vi "WildBugChilGru_V2.0.0.vi"() -> ()   [LabVIEW 2014]
uses:
  <vilib>/Utility/miscctls.llb/LVPointTypeDef.ctl
  <vilib>/Utility/xml.llb/Read From XML File(string).vi
  <vilib>/Utility/xml.llb/Write to XML File(string).vi
  <vilib>/Instr/_visa.llb/VISA Configure Serial Port (Instr).vi
  <vilib>/Analysis/3filter.llb/IIR Filter (DBL).vi
  <vilib>/gmath/NI_Gmath.lvlib
  <vilib>/Analysis/NI_AALBase.lvlib
panel:
  in  "Registerkarte":T1(tab)
  in  "Zündung [Imp/U]":dbl=1.0
  in  "Übersetzung ermitteln aus":T2(ring)
  in  "Getriebe [1:]":dbl=5.343
  in  "Reifenumfang [m]":dbl=1.222
  in  "Dauer [s]":dbl=5.0
  in  "nKuWe/nRolle":dbl=10.0
  in  "Lufttemperatur [°C]":dbl=20.0
  in  "Luftfeuchtigkeit [%]":dbl=50.0
  in  "Luftdruck [mbar]":dbl=1013.0
  in  "Messung Klimadaten":bool=TRUE
  in  "Gleitender Mittelwert":u8=35
  in  "Differenzenquotient":u8=12
  in  "n vom Gas [1/min]":dbl=5000.0
  in  "Rollengeber [Inkr/U]":u16=200
  in  "Rollenumfang [m]":dbl=0.613
  in  "Rollenträgheit [kgm²]":dbl=0.402
  in  "Recalc":bool
  in  "Ende":bool
  out "Datenspeicher":T3={"Fahrzeugdaten"="", "date/time string"="", "Rolle [Inkr/U]"=0, "Rollenumfang [m]"=0.0, "Rollenträgheit [kgm²]"=0.0, "Zündung [Imp/U]"=0.0, "Getriebe [1:]"=0.0, "Reifenumfang [m] "=0.0, "element"=0.0, "Gl. Mittelwert"=0, "Differenzenquotient"=0, "Polynom"=0, "dT [s]"=0.0, "element"=0.0, "Lufttemperatur [°C]"=0.0, "Luftfeuchtigkeit [%]"=0.0, "Luftdruck [mbar]"=0.0, [], [], "Best Polynomial Fit"=[], [], "Übersetzung ermitteln aus"=0, "[s]"=0.0, "nmin [1/min]"=0.0, "nmax [1/min]"=0.0, "n vom Gas [1/min]"=0.0, "dT-Array [s]"=[], [], "Boolesch"=FALSE, "Serielle Schnittstelle"="COM4", "nKuWe/nRolle"=10.0}
  out "COM-Fehlerrate":string="0 / 0,0%"
  in  "Konfiguration:":bool
  in  "Speichern":bool
  in  "Drucken":bool
  out "Pmax":string="0,0 PS"
  out "Ergebnis":string="0,0 PS bei 0 1/min   |   0,0 Nm bei 0 1/min   |   vmax: 2147483647 km/h\nDIN 70020 k =1,000 (20 °C, 50 %, 1013 mbar)\n20.11.2016 20:05 "
  in  "Fahrzeugdaten":string="Hier die Fahrzeugdaten eingeben"
  out "XY-Graph":cluster{dbl[], dbl[]}[](graph)
  out "Untersetzung\nermittelt":bool
  out "Untersetzung":dbl format="%#.2f"
  in  "Start":bool
  out "Füllstand Lesepuffer":u64(slide) scale=1.0..100.0
  out "Hinterrad\n[km/h]":dbl(knob) scale=0.0..150.0
  out "Welle\n[1/min]":cluster{dbl, dbl}(knob) scale=0.0..14000.0
  out "Lesepuffer":string="\n"
  in  "Serielle Schnittstelle":refnum<visa-resource-name>="COM4"
  out "Untersetzung-Graph":dbl(graph)=2.6802446808510636 caption="Untersetzung"
  # "1. n konstant halten\n2. START\n3. n weiter halten\n4. bei GO: Vollgas\n5. vom Gas gehen"
  # "Zündung\nRolle"
  # "Untersetzung aus:"
  # "Eingabe <> Messen"
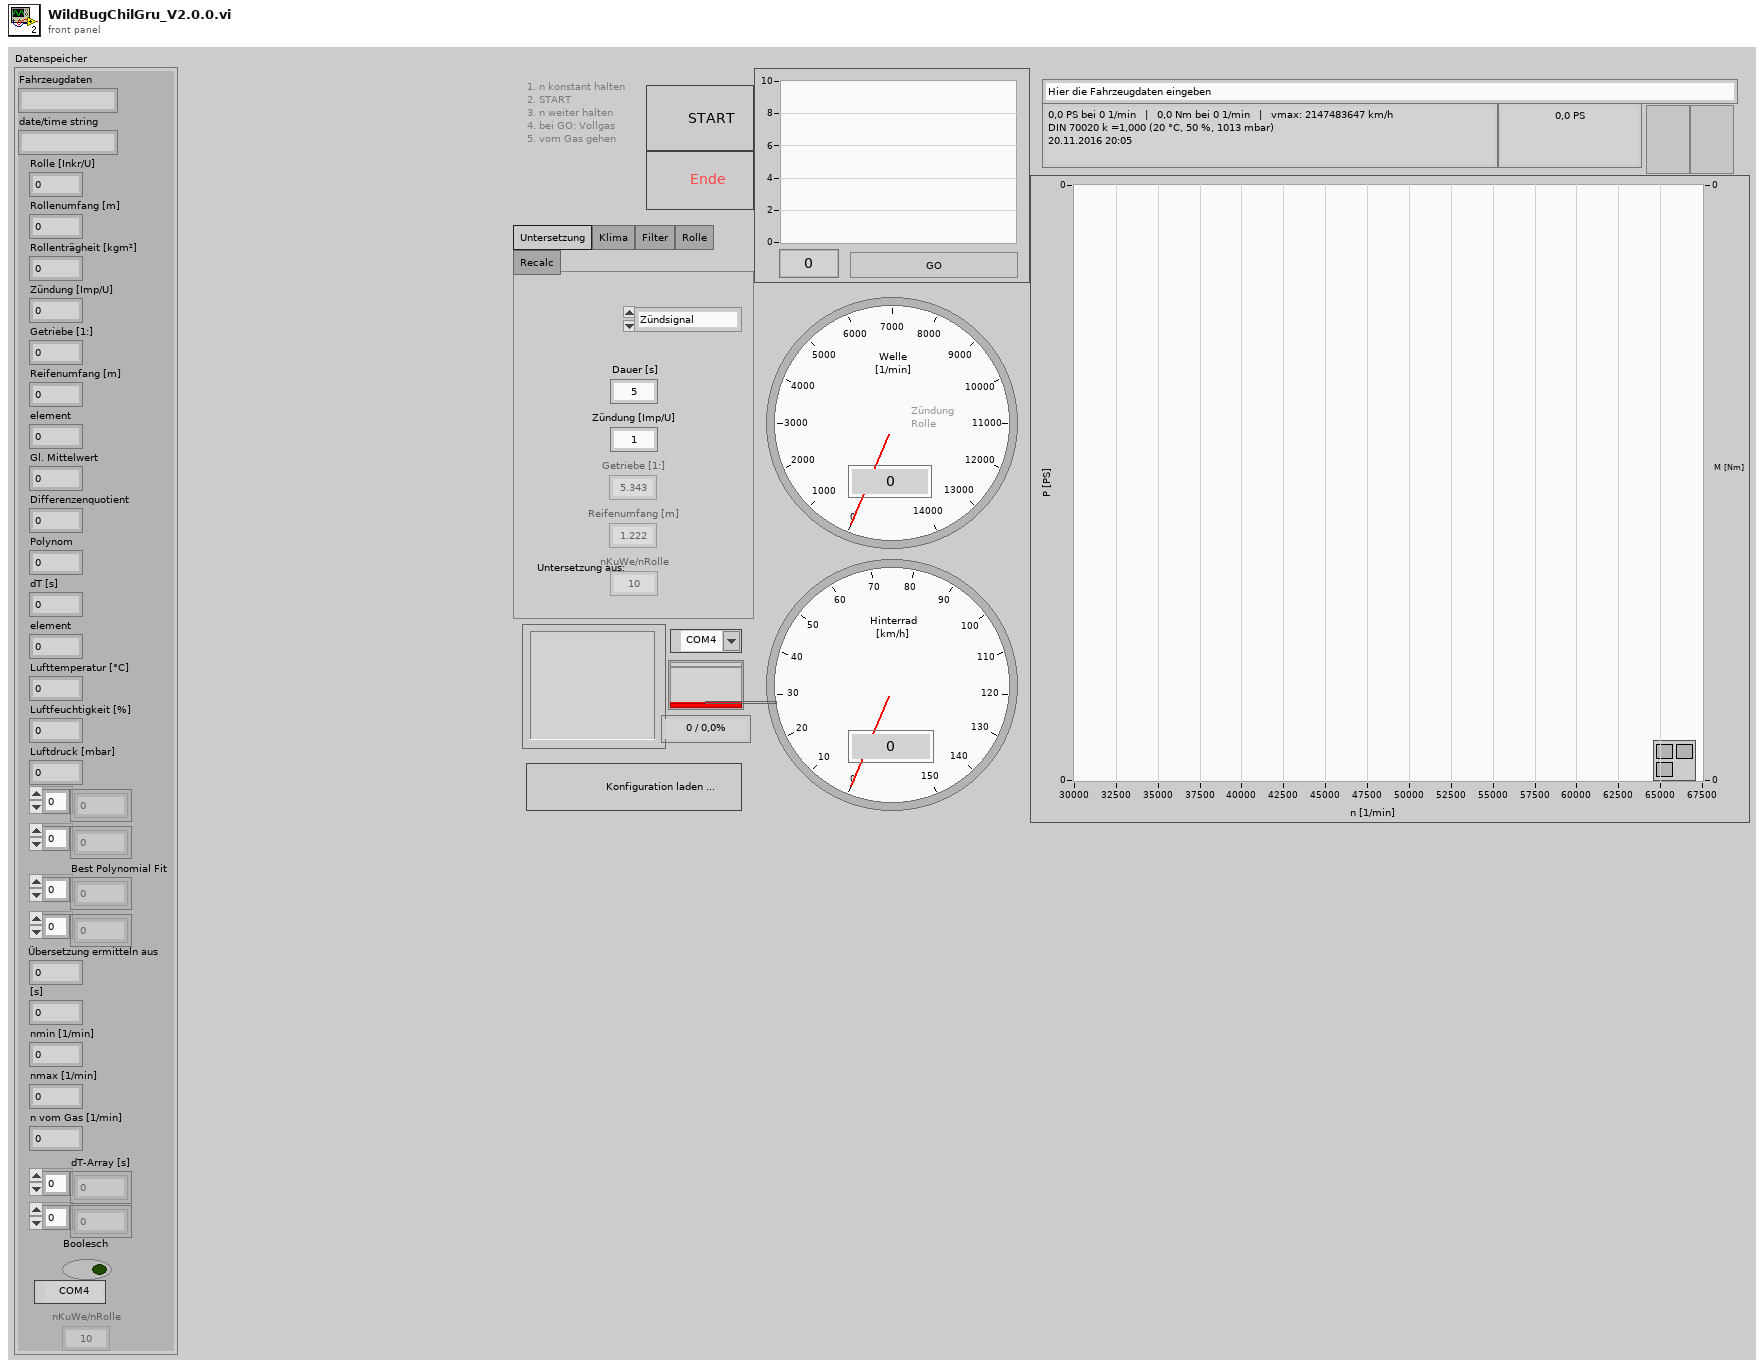
[diagram p1: front panel]
types:
  T1 = enum32{"Untersetzung", "Klima", "Filter", "Rolle", "Recalc"}
  T2 = enum8{"Zündsignal", "Getriebe & Reifen", "nKuWe / nRolle"}
  T3 = cluster{"Fahrzeugdaten":string, "date/time string":string, "Rolle [Inkr/U]":u16, "Rollenumfang [m]":dbl, "Rollenträgheit [kgm²]":dbl, "Zündung [Imp/U]":dbl, "Getriebe [1:]":dbl, "Reifenumfang [m] ":dbl, "element":dbl, "Gl. Mittelwert":u8, "Differenzenquotient":u8, "Polynom":u8, "dT [s]":dbl, "element":dbl, "Lufttemperatur [°C]":dbl, "Luftfeuchtigkeit [%]":dbl, "Luftdruck [mbar]":dbl, dbl[], dbl[], "Best Polynomial Fit":dbl[], dbl[], "Übersetzung ermitteln aus":u8, "[s]":dbl, "nmin [1/min]":dbl, "nmax [1/min]":dbl, "n vom Gas [1/min]":dbl, "dT-Array [s]":dbl[], i32[], "Boolesch":bool, "Serielle Schnittstelle":refnum<visa-resource-name>, "nKuWe/nRolle":dbl}
  T4 = enum8{"Enabled", "Disabled", "Disabled and Grayed Out"}
  T5 = cluster{"Fahrzeugdaten":string, "date/time string":string, "Rollengeber [Inkr/U]":u16, "Rollenumfang [m]":dbl, "Rollenträgheit [kgm²]":dbl, "Zündung [Imp/U]":dbl, "Getriebe [1:]":dbl, "Reifenumfang [m] ":dbl, "mean value":dbl, "Gleitender Mittelwert":u8, "Differenzenquotient":u8, i32, dbl, "element":dbl, "Lufttemperatur [°C]":dbl, "Luftfeuchtigkeit [%]":dbl, "Luftdruck [mbar]":dbl, dbl[], dbl[], dbl[], dbl[], "Übersetzung ermitteln aus":enum8{"Zündsignal", "Getriebe & Reifen", "nKuWe / nRolle"}, "Dauer [s]":dbl, dbl, dbl, "n vom Gas [1/min]":dbl, dbl[], i32[], "Messung Klimadaten":bool, "VISA resource name out":refnum<visa-resource-name>, "nKuWe/nRolle":dbl}
  T6 = cluster{"Fahrzeugdaten":string, "date/time string":string, "Rolle [Inkr/U]":u16, "Rollenumfang [m]":dbl, "Rollenträgheit [kgm²]":dbl, "Zündung [Imp/U]":dbl, "Getriebe [1:]":dbl, "Reifenumfang [m] ":dbl, "element":dbl, "Gl. Mittelwert":u8, "Differenzenquotient":u8, "Polynom":u8, "element":dbl, "element":dbl, "Lufttemperatur [°C]":dbl, "Luftfeuchtigkeit [%]":dbl, "Luftdruck [mbar]":dbl, dbl[], dbl[], "Best Polynomial Fit":dbl[], dbl[], "Übersetzung ermitteln aus":u8, "[s]":dbl, "nmin [1/min]":dbl, "nmax [1/min]":dbl, "n vom Gas [1/min]":dbl, dbl[], i32[], "Boolesch":bool, "Serielle Schnittstelle":refnum<visa-resource-name>, dbl}
  T7 = typedef "LVPointTypeDef.ctl" = cluster{"Horizontal":i16, "Vertical":i16}
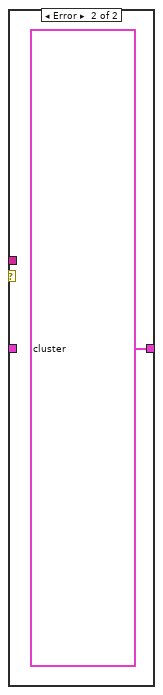
[diagram p2: hidden frame]
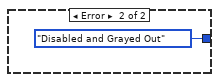
[diagram p3: hidden frame]
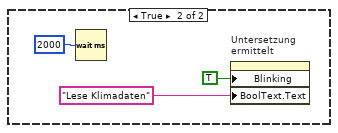
[diagram p5: hidden frame]
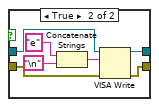
[diagram p6: hidden frame]
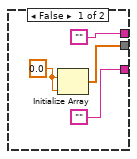
[diagram p8: hidden frame]
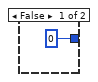
[diagram p10: hidden frame]
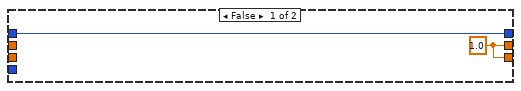
[diagram p12: hidden frame]
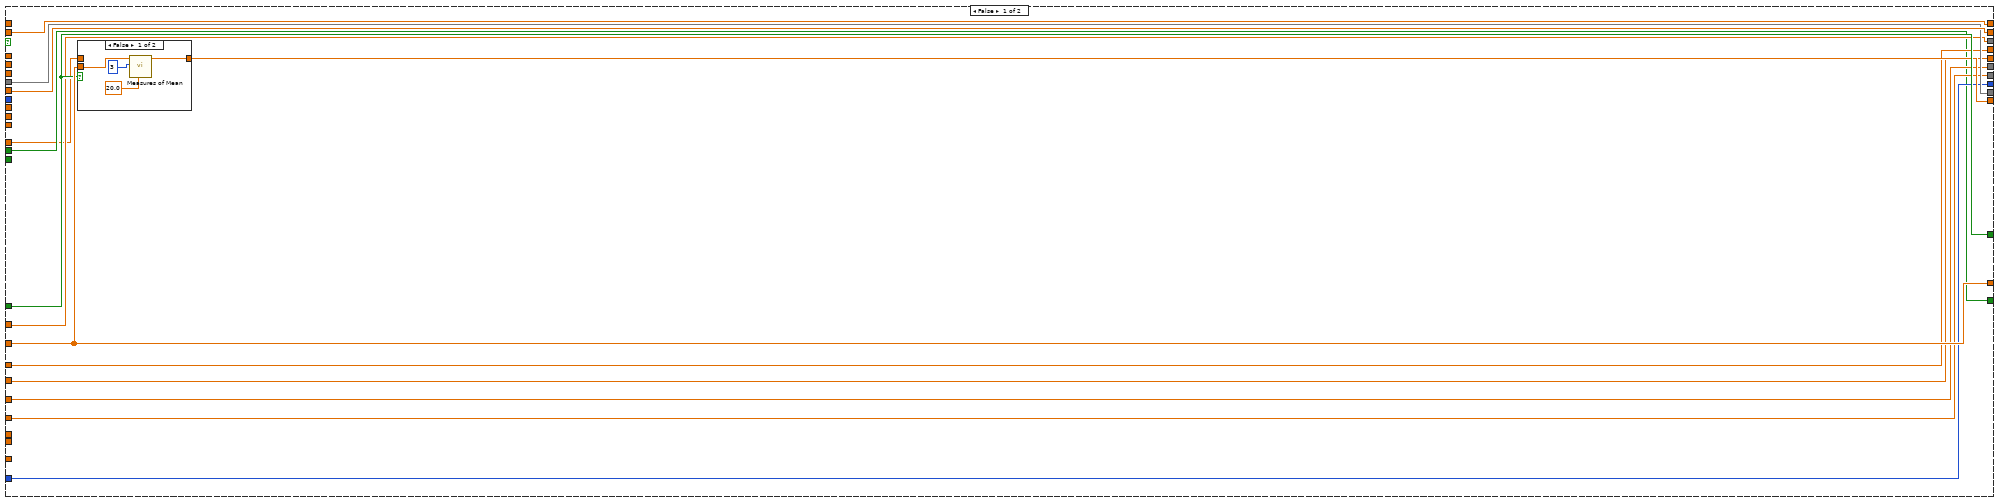
[diagram p13: hidden frame]
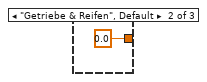
[diagram p17: hidden frame]
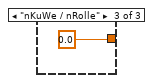
[diagram p18: hidden frame]
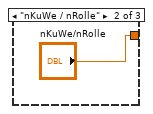
[diagram p20: hidden frame]
diagram:
  n1 = while {
    stop <- w1 stop-if-true
    n2 = local read "Start"() -> (w2:bool)
    n3 = case shown="True" w2 {
      frame False {
      }
      frame True {
        n4 = flat-sequence {
          tunnel: [w128] -> w116
          tunnel: [w127] -> w115
          tunnel: ["Messung Klimadaten"] -> w114
          tunnel: w116 -> [w141]
          tunnel: w115 -> [w140]
          tunnel: [0] -> w113
          tunnel: [1.0 ("element")] -> w112
          tunnel: [w138] -> w111
          tunnel: [w152] -> w110
          tunnel: [0] -> w109
          tunnel: [w138] -> w108
          tunnel: [-5] -> w107
          tunnel: [w149] -> w106
          tunnel: [w147] -> w105
          tunnel: [w146] -> w104
          tunnel: [0.0] -> w103
          tunnel: [w141] -> w102
          tunnel: [w140] -> w101
          tunnel: w114 -> [w139]
          tunnel: [w139] -> w100
          tunnel: w113 -> [w178]
          tunnel: [w178] -> w99
          tunnel: w112 -> [w177]
          tunnel: [w177] -> w98
          tunnel: w111 -> [w176]
          tunnel: [w176] -> w97
          tunnel: w110 -> [w175]
          tunnel: [w175] -> w96
          tunnel: w109 -> [w174]
          tunnel: [w174] -> w95
          tunnel: w108 -> [w173]
          tunnel: [w173] -> w94
          tunnel: w107 -> [w172]
          tunnel: [w172] -> w93
          tunnel: w106 -> [w171]
          tunnel: [w171] -> w92
          tunnel: w105 -> [w170]
          tunnel: [w170] -> w91
          tunnel: w104 -> [w169]
          tunnel: [w169] -> w90
          tunnel: w103 -> [w168]
          tunnel: [w168] -> w89
          tunnel: w102 -> [w167]
          tunnel: [w164] -> w88
          tunnel: w101 -> [w166]
          tunnel: [w165] -> w87
          tunnel: [w163] -> w86
          tunnel: w100 -> [w163]
          tunnel: w99 -> [w202]
          tunnel: [w202] -> w85
          tunnel: w98 -> [w201]
          tunnel: [w201] -> w84
          tunnel: w97 -> [w200]
          tunnel: [w200] -> w83
          tunnel: w96 -> [w199]
          tunnel: [w199] -> w82
          tunnel: w95 -> [w198]
          tunnel: [w198] -> w81
          tunnel: w94 -> [w197]
          tunnel: [w197] -> w80
          tunnel: w93 -> [w196]
          tunnel: [w196] -> w79
          tunnel: w92 -> [w195]
          tunnel: [w195] -> w78
          tunnel: w91 -> [w194]
          tunnel: [w194] -> w77
          tunnel: w90 -> [w193]
          tunnel: [w193] -> w76
          tunnel: w89 -> [w192]
          tunnel: [w192] -> w75
          tunnel: w88 -> [w191]
          tunnel: [w191] -> w74
          tunnel: w87 -> [w190]
          tunnel: [w190] -> w73
          tunnel: w86 -> [w188]
          tunnel: [w188] -> w72
          tunnel: w85 -> [w218]
          tunnel: [w218] -> w71
          tunnel: w84 -> [w217]
          tunnel: [w217] -> w70
          tunnel: w83 -> [w216]
          tunnel: [w216] -> w69
          tunnel: w82 -> [w215]
          tunnel: [w215] -> w68
          tunnel: w81 -> [w214]
          tunnel: [w214] -> w67
          tunnel: w80 -> [w213]
          tunnel: [w213] -> w66
          tunnel: w79 -> [w212]
          tunnel: [w212] -> w65
          tunnel: w78 -> [w211]
          tunnel: [w211] -> w64
          tunnel: w77 -> [w210]
          tunnel: [w210] -> w63
          tunnel: w76 -> [w209]
          tunnel: [w209] -> w62
          tunnel: w75 -> [w208]
          tunnel: [w208] -> w61
          tunnel: w74 -> [w207]
          tunnel: [w206] -> w60
          tunnel: w73 -> [w204]
          tunnel: [w205] -> w59
          tunnel: w72 -> [w203]
          tunnel: w71 -> [w297]
          tunnel: w70 -> [w296]
          tunnel: w69 -> [w295]
          tunnel: w68 -> [w294]
          tunnel: w67 -> [w293]
          tunnel: w66 -> [w292]
          tunnel: w65 -> [w291]
          tunnel: w64 -> [w290]
          tunnel: w63 -> [w289]
          tunnel: w62 -> [w288]
          tunnel: w61 -> [w287]
          tunnel: w60 -> [w253]
          tunnel: [w297] -> w58
          tunnel: [w296] -> w57
          tunnel: [w295] -> w56
          tunnel: [w294] -> w55
          tunnel: [w293] -> w54
          tunnel: [w292] -> w53
          tunnel: [w291] -> w52
          tunnel: [w290] -> w51
          tunnel: [w289] -> w50
          tunnel: [w288] -> w49
          tunnel: [w287] -> w48
          tunnel: [w253] -> w47
          tunnel: [w252] -> w46
          tunnel: [w286] -> w45
          tunnel: [w285] -> w44
          tunnel: [w284] -> w43
          tunnel: ["Gleitender Mittelwert"] -> w42
          tunnel: w59 -> [w252]
          tunnel: [w246] -> w5
          tunnel: [w245] -> w4
          tunnel: [w306] -> w14
          tunnel: [w307] -> w15
          tunnel: [w308] -> w16
          tunnel: [w309] -> w17
          tunnel: [w300] -> w12
          tunnel: [w299] -> w13
          tunnel: [w310] -> w18
          tunnel: [w311] -> w19
          tunnel: [w312] -> w21
          tunnel: [w313] -> _
          tunnel: [w314] -> w23
          tunnel: [w315] -> w24
          tunnel: [w316] -> w37
          tunnel: [w317] -> w3
          tunnel: [w318] -> w39
          tunnel: [w319] -> w40
          tunnel: [w320] -> w41
          tunnel: w58 -> [w320]
          tunnel: w57 -> [w319]
          tunnel: w56 -> [w318]
          tunnel: w55 -> [w317]
          tunnel: w54 -> [w316]
          tunnel: w53 -> [w315]
          tunnel: w52 -> [w314]
          tunnel: w51 -> [w313]
          tunnel: w50 -> [w312]
          tunnel: w49 -> [w311]
          tunnel: w48 -> [w310]
          tunnel: w47 -> [w302]
          tunnel: w46 -> [w301]
          tunnel: w45 -> [w309]
          tunnel: w44 -> [w308]
          tunnel: w43 -> [w307]
          tunnel: w42 -> [w306]
          frame #0 {
            w133 = u16 0 items=["None", "XON/XOFF", "RTS/CTS", "XON/XOFF & RTS/CTS", "DTR/DSR", "XON/XOFF & DTR/DSR"] ("flow control (0:none)")
            w134 = u16 10 items=["1.0"=10, "1.5"=15, "2.0"=20] ("stop bits (10: 1 bit)")
            w126 = FALSE  # Enable Termination Char (T)
            w129 = u32 10000  # timeout (10sec)
            n5 = call-poly "VISA Configure Serial Port"("VISA resource name"="Serielle Schnittstelle", "timeout (10sec)"=w129, "Enable Termination\nChar (T)"=w126, "baud rate (9600)"=u32 115200 ("baudrate (250000)"), "data bits (8)"=u16 8, "parity (0:none)"=enum16{"None", "Odd", "Even", "Mark", "Space"}."None", "stop bits (10: 1 bit)"=w134, "flow control (0:none)"=w133) -> ("VISA resource name out"=w131:refnum<visa-resource-name>, "error out"=w130:errorcluster)  [unwired: 6 in]
            n6 = VISA Clear(VISA resource name=w131, error in (no error)=w130) -> (VISA resource name out=w128:refnum<visa-resource-name>, error out=w127:errorcluster)
          }
          frame #1 {
            w142 = T4."Disabled and Grayed Out" ("Deaktiviert")
            w145 = 0.0  # Graphen löschen
            w148 = 0
            w153 = 0.0
            w138 = FALSE
            w146 = ""
            n7 = case shown="False" w139 {
              frame False {
                n8 = property on="Untersetzung\nermittelt" class="Bool. (strikt)"("Blinking"=TRUE ("Blinkend"), "BoolText.Text"="Initialisiere" ("Beschriftung.Text")) -> ()  [unwired: 2 in, 2 out]
              }
              frame True {
                n9 = Wait (ms)(milliseconds to wait=u32 2000 ("Zu wartende ms")) -> ()  [unwired: 1 out]
                n10 = property on="Untersetzung\nermittelt" class="Bool. (strikt)"("Blinking"=TRUE ("Blinkend"), "BoolText.Text"="Lese Klimadaten" ("Beschriftung.Text")) -> ()  [unwired: 2 in, 2 out]
              }
            }
            n11 = Build Array(w145) -> (w144:dbl[])
            n12 = property on="Drucken" class="Bool. (strikt)"("DisabledEnum"=w142) -> ()  [unwired: 2 in, 2 out]
            n13 = property on="Übersetzung ermitteln aus" class="Enum (strikt)"("DisabledEnum"=w142) -> ()  [unwired: 2 in, 2 out]
            n14 = property on="Konfiguration:" class="Bool. (strikt)"("DisabledEnum"=w142) -> ()  [unwired: 2 in, 2 out]
            n15 = property on="Ende" class="Bool. (strikt)"("DisabledEnum"=w142) -> ()  [unwired: 2 in, 2 out]
            n16 = property on="Speichern" class="Bool. (strikt)"("DisabledEnum"=w142) -> ()  [unwired: 2 in, 2 out]
            n17 = property on="Untersetzung-Graph" class="SVDiagr (strikt)"("History Data"=w144) -> ()  [unwired: 2 in, 2 out]
            n18 = local write "Pmax"(w146) -> ()
            n19 = local write "COM-Fehlerrate"(w146) -> ()
            n20 = local write "Ergebnis"(w146) -> ()
            n21 = Initialize Array(w153, w153) -> (w152:dbl[])
            n22 = Initialize Array(0.0 ("y"), 0) -> (w149:dbl[])
            n23 = Initialize Array(w148, w148) -> (w147:i32[])
          }
          frame #2 {
            n24 = case shown="False" w163 {
              tunnel: w167 -> [w180 w184]
              tunnel: w166 -> [w179 w183]
              tunnel: [w179 w182] -> w165
              tunnel: [w180 w181] -> w164
              frame False {
              }
              frame True {
                n25 = Concatenate Strings("e" ("String"), "\n") -> (w187:string)
                n26 = VISA Write(VISA resource name=w184, write buffer=w187, error in (no error)=w183) -> (VISA resource name out=w181:refnum<visa-resource-name>, error out=w182:errorcluster)  [unwired: 1 out]
              }
            }
          }
          frame #3 {
            n27 = Wait (ms)(milliseconds to wait=u32 500 ("Zu wartende ms")) -> ()  [unwired: 1 out]
          }
          frame #4 {
            n28 = case shown="True" w203 {
              tunnel: w207 -> [w220 w241]
              tunnel: [w220 w240] -> w206
              tunnel: [w219 w239] -> w205
              tunnel: w204 -> [w219 w238]
              frame False {
              }
              frame True {
                w223 = ";" ("Regulärer Ausdruck")
                n29 = property class="Instr"(reference=w241, error in=w238) -> (reference out=w244:refnum<visa-resource-name>, error out=w243:errorcluster, "Serial Settings:Number of Bytes at Serial Port"=w242:u32)
                n30 = VISA Read(VISA resource name=w244, byte count=w242, error in (no error)=w243) -> (VISA resource name out=w240:refnum<visa-resource-name>, read buffer=w235:string, error out=w239:errorcluster)  [unwired: 1 out]
                n31 = Search and Replace String(replace all?=TRUE ("Alle ersetzen? (F)"), input string=w235, search string="." ("Such-String"), replace string="," ("Ersetzungs-String (\"\")")) -> (result string=w228:string)  [unwired: 4 in, 3 out]
                n32 = Match Pattern(string=w228, regular expression=w223) -> (before substring=w226:string, after substring=w227:string)  [unwired: 1 in, 2 out]
                n33 = Match Pattern(string=w227, regular expression=w223) -> (before substring=w225:string, after substring=w224:string)  [unwired: 1 in, 2 out]
                n34 = Fract/Exp String To Number(string=w226, offset=0 ("Offset")) -> (number=w234:dbl)  [unwired: 2 in, 1 out]
                n35 = local write "Lufttemperatur [°C]"(w234) -> ()
                n36 = Fract/Exp String To Number(string=w225) -> (number=w231:dbl)  [unwired: 3 in, 1 out]
                n37 = Match Pattern(string=w224, regular expression=w223) -> (before substring=w222:string)  [unwired: 1 in, 3 out]
                n38 = Fract/Exp String To Number(string=w222) -> (number=w233:dbl)  [unwired: 3 in, 1 out]
                n39 = Divide(x=w231, y=100.0 ("x")) -> (x/y=w232:dbl)
                n40 = local write "Luftdruck [mbar]"(w232) -> ()
                n41 = local write "Luftfeuchtigkeit [%]"(w233) -> ()
              }
            }
          }
          frame #5 {
            n42 = Wait (ms)(milliseconds to wait=u32 2000 ("Zu wartende ms")) -> ()  [unwired: 1 out]
            n43 = Add(x="Lufttemperatur [°C]", y=273.15) -> (x+y=w268:dbl)
            n44 = Divide ("M_Welle [Nm]")(x=300.0, y=w268) -> (x/y=w271:dbl)
            n45 = Multiply(x="Luftfeuchtigkeit [%]", y=0.01) -> (x*y=w281:dbl)
            n46 = Divide ("M_Welle [Nm]")(x=w268, y=293.15) -> (x/y=w266:dbl)
            n47 = Multiply(x=w281, y=240800000000.0) -> (x*y=w256:dbl)
            n48 = Power Of X(1:w271, 2:5.0) -> (0:w269:dbl)
            n49 = Multiply(x=w256, y=w269) -> (x*y=w275:dbl)
            n50 = Multiply(x=w271, y=-22.644) -> (x*y=w276:dbl)
            n51 = Power Of X(1:w266, 2:0.5) -> (0:w263:dbl)
            n52 = Exponential(1:w276) -> (0:w274:dbl)
            n53 = Multiply "Dampfdruck"(x=w275, y=w274) -> ()  [unwired: 1 out]
            n54 = Subtract "Bei DIN70200 ist absoluter Druck zu verwenden,\nohne Damprdruck abzuziehen!"(x="Luftdruck [mbar]", y=0.0) -> (x-y=w272:dbl)
            n55 = local read "Differenzenquotient"() -> (w247:u8)
            n56 = Divide ("M_Welle [Nm]")(x=1013.0, y=w272) -> (x/y=w264:dbl)
            n57 = Multiply "Korrekturfaktor DIN 70020"(x=w264, y=w263) -> (x*y=w286:dbl)
            n58 = Divide(x="Gleitender Mittelwert", y=2) -> (x/y=w260:dbl)
            n59 = call <vilib>:"Smoothing Filter Coefficients.vi"("shape"=0, "half-width"=w247, "type"=0) -> ("forward coefficients"=w245:dbl[], "reverse coefficients"=w246:dbl[])  [unwired: 6 in, 1 out]
            n60 = Round Toward -Infinity(1:w260) -> (0:w259:dbl)
            n61 = call <vilib>:"Smoothing Filter Coefficients.vi"("shape"=1, "half-width"=w259, "type"=0) -> ("forward coefficients"=w284:dbl[], "reverse coefficients"=w285:dbl[])  [unwired: 6 in, 1 out]
          }
          frame #6 {
            n62 = Concatenate Strings("m" ("String"), "\n") -> (w305:string)
            n63 = property on="Untersetzung\nermittelt" class="Bool. (strikt)"("Blinking"=FALSE ("Blinkend")) -> ()  [unwired: 2 in, 2 out]
            n64 = VISA Write(VISA resource name=w302, write buffer=w305, error in (no error)=w301) -> (VISA resource name out=w299:refnum<visa-resource-name>, error out=w300:errorcluster)  [unwired: 1 out]
          }
        }
        n65 = while {
          tunnel: w13 -> [w438]
          tunnel: w12 -> [w437]
          shift-right: [w504] -> _
          shift-left: w19 -> [w453]
          shift-right: [w499] -> _
          shift-left: w18 -> [w503]
          shift-right: [w498] -> _
          shift-left: w18 -> [w502]
          shift-right: [w457] -> _
          shift-left: w18 -> [w501]
          shift-right: [w483] -> _
          shift-left: w41 -> [w500]
          shift-right: [w445] -> w26
          shift-left: w40 -> [_]
          shift-right: [w462] -> w30
          shift-left: w18 -> [w432]
          shift-right: [w427] -> w28
          shift-left: w18 -> [w459]
          shift-right: [w458] -> _
          shift-left: _ -> [w495]
          shift-right: [w430] -> _
          shift-left: w39 -> [w472]
          shift-right: [w439] -> _
          shift-left: w3 -> [_]
          shift-right: [w444] -> _
          shift-left: w3 -> [_]
          shift-right: [w492] -> w29
          shift-left: w3 -> [w490]
          shift-right: [w491] -> _
          shift-left: w3 -> [w489]
          shift-right: [w478] -> w36
          shift-left: _ -> [w488]
          shift-right: [w482] -> _
          shift-left: _ -> [w486]
          shift-right: [w481] -> w6
          shift-left: _ -> [w487]
          shift-right: [w480] -> w35
          shift-left: _ -> [w485]
          shift-right: [w479] -> w34
          shift-left: _ -> [w484]
          tunnel: [w477] -> w38
          shift-right: [w473] -> w33
          shift-left: w37 -> [w475]
          tunnel: [w476] -> w9
          tunnel: ["n vom Gas [1/min]"] -> w32
          tunnel: ["Rollenumfang [m]"] -> w31
          tunnel: ["Rollenumfang [m]"] -> w25
          shift-right: [w469] -> _
          shift-left: w24 -> [w436]
          shift-right: [w463] -> _
          shift-left: w23 -> [w468]
          shift-right: [w464] -> _
          shift-left: w18 -> [w467]
          shift-right: [w465] -> _
          shift-left: w18 -> [w466]
          shift-right: [w435] -> w22
          shift-left: w3 -> [w461]
          shift-right: [w456] -> _
          shift-left: _ -> [w455]
          shift-right: [w460] -> w20
          shift-left: w21 -> [w454]
          tunnel: [w452] -> w10
          tunnel: w17 -> [w445]
          tunnel: w16 -> [w439]
          tunnel: w15 -> [w444]
          tunnel: w14 -> [w443]
          tunnel: w5 -> [w434]
          tunnel: w4 -> [w433]
          stop <- w477 stop-if-true
          n66 = property class="Instr"(reference=w438, error in=w437) -> (reference out=w448:refnum<visa-resource-name>, error out=w447:errorcluster, "Serial Settings:Number of Bytes at Serial Port"=w450:u32)
          n67 = Greater?(x=w450, y=u32 1 ("min. Bytes")) -> (0:w446:bool)
          n68 = case shown="True" w446 {
            tunnel: w450 -> [_ w507]
            tunnel: [u32 0 ("Bytes at Port") w507] -> w449
            frame False {
            }
            frame True {
            }
          }
          n69 = case shown="1.." w449 {
            selector: w449 -> [_ w773]
            tunnel: [w723 w767] -> w476
            tunnel: [w722 w768] -> w452
            tunnel: [w727 w769] -> w498
            tunnel: [w728 w766] -> w499
            tunnel: w453 -> [w729 w764]
            tunnel: [w729 w762] -> w504
            tunnel: w503 -> [w728 w754]
            tunnel: w502 -> [w727 w753]
            tunnel: [w724 w752] -> w457
            tunnel: w501 -> [w724 w751]
            tunnel: w500 -> [w726 _]
            tunnel: [w726 w734] -> w483
            tunnel: [w725 w740] -> w456
            tunnel: w455 -> [w725 w739]
            tunnel: w448 -> [w722 w731]
            tunnel: w447 -> [w723 w730]
            frame 0, Default {
              # "No data in from serial port - Nothing to do."
            }
            frame 1.. {
              # "Hz Drum"
              n70 = VISA Read(VISA resource name=w731, byte count=w773, error in (no error)=w730) -> (VISA resource name out=w768:refnum<visa-resource-name>, read buffer=w765:string, error out=w767:errorcluster)  [unwired: 1 out]
              n71 = Concatenate Strings(w764, w765) -> (w736:string)
              "Lesepuffer" <- w736
              n72 = Spreadsheet String To Array(delimiter (Tab)="\n" ("regular expression"), format string="%s" ("regular expression"), spreadsheet string=w736, array type (2D Dbl)=string[] [] ("Array 2")) -> (array=w745:string[])
              n73 = Match Pattern(string=w736, regular expression="[\\n]") -> (before substring=w743:string, after substring=w763:string, offset past match=w777:i32)  [unwired: 1 in, 1 out]
              n74 = Array Size(array=w745) -> (size(s)=w749:i32)
              n75 = Match Pattern(string=w743, regular expression="[;]") -> (before substring=w741:string, after substring=w742:string, offset past match=w738:i32)  [unwired: 1 in, 1 out]
              n76 = Subtract "aktuelle Zeilenanzahl"(x=w749, y=1) -> (x-y=w734:i32)
              n77 = property on="Füllstand Lesepuffer" class="Schieber (strikt)"() -> ("Scale.Maximum"=w733:dbl)  [unwired: 2 in, 2 out]
              n78 = Match Pattern(string=w742, regular expression="[;]") -> (before substring=w772:string, after substring=w775:string, offset past match=w760:i32)  [unwired: 1 in, 1 out]
              n79 = Match Pattern(string=w775, regular expression="[;]") -> (before substring=w771:string, after substring=w770:string, offset past match=w758:i32)  [unwired: 1 in, 1 out]
              n80 = Greater Or Equal To 0?(x=w738) -> (x >= 0?=w737:bool)
              n81 = Greater?(x=w734, y=w733) -> (0:w735:bool)
              n82 = Greater Or Equal To 0?(x=w758) -> (x >= 0?=w757:bool)
              n83 = Greater Or Equal To 0?(x=w760) -> (x >= 0?=w759:bool)
              n84 = Greater Or Equal To 0?(x=w777) -> (x >= 0?=w761:bool)
              n85 = Select(t=w734, s=w735, f=w733) -> (s? t:f=w732:dbl)
              n86 = Build Array(w761, w759, w737, w757) -> (w756:bool[])
              n87 = property on="Füllstand Lesepuffer" class="Schieber (strikt)"("Scale.Maximum"=w732) -> ()  [unwired: 2 in, 2 out]
              n88 = And Array Elements(Boolean array=w756) -> (logical AND=w755:bool)
              n89 = case shown="True" w755 {
                tunnel: w772 -> [_ w788]
                tunnel: w771 -> [_ w793]
                tunnel: w770 -> [_ w792]
                tunnel: [w781 w791] -> w769
                tunnel: [w782 w790] -> w766
                tunnel: w763 -> [_ w789]
                tunnel: [w783 w789] -> w762
                tunnel: w736 -> [w783 _]
                tunnel: w754 -> [w782 _]
                tunnel: w753 -> [w781 _]
                tunnel: [w780 w787] -> w752
                tunnel: w751 -> [w780 _]
                tunnel: w741 -> [_ w786]
                tunnel: [w779 w784] -> w740
                tunnel: w739 -> [w779 _]
                frame False {
                }
                frame True {
                  # "Cyclecounter"
                  # "Hz ComLevel"
                  # "ComLevel\nLevel 10 =   6Hz \nLevel 5 =   12Hz \nLevel 4 =   15Hz\nLevel 3 =   20Hz\nLevel 2 =   33Hz\nLevel 1 =   62Hz"
                  # "Hz Drum"
                  # "Hz Engine"
                  # "t4m"
                  n90 = Fract/Exp String To Number(string=w786) -> (number=w785:dbl)  [unwired: 3 in, 1 out]
                  n91 = Fract/Exp String To Number(string=w792) -> (number=w791:dbl)  [unwired: 3 in, 1 out]
                  n92 = Fract/Exp String To Number(string=w788) -> (number=w787:dbl)  [unwired: 3 in, 1 out]
                  n93 = To Long Integer(number=w785) -> (32bit integer=w784:i32)
                  n94 = Fract/Exp String To Number(string=w793) -> (number=w790:dbl)  [unwired: 3 in, 1 out]
                }
              }
            }
          }
          "Füllstand Lesepuffer" <- w483
          n95 = Not Equal?(x=w455, y=w456) -> (x != y?=w440:bool)
          n96 = case shown="True" w440 {
            tunnel: w468 -> [w511 w522]
            tunnel: [w511 w534] -> w463
            tunnel: w467 -> [w510 w533]
            tunnel: [w510 w519] -> w464
            tunnel: w466 -> [w509 w532]
            tunnel: [w509 w520] -> w465
            tunnel: w456 -> [_ w518]
            tunnel: w454 -> [w508 w517]
            tunnel: [w508 w521] -> w460
            frame False {
            }
            frame True {
              n97 = Build Array (concatenate)(w517, w518) -> (w521:i32[])
              n98 = Greater Or Equal To 0?(x=w522) -> (x >= 0?=w523:bool)
              n99 = case shown="True" w523 {
                tunnel: [w535 w546] -> w519
                tunnel: [w535 w547] -> w520
                tunnel: [w536 w538] -> w534
                tunnel: w533 -> [_ w540]
                tunnel: w532 -> [_ w548]
                tunnel: w518 -> [w536 w537]
                tunnel: w522 -> [_ w538]
                frame False {
                  w535 = 1.0
                }
                frame True {
                  w544 = 65536.0
                  n100 = Add(x=w538, y=w540) -> (x+y=w539:dbl)
                  n101 = Increment(x=w548) -> (x+1=w547:dbl)
                  n102 = Divide(x=w539, y=w544) -> (x/y=w549:dbl)
                  n103 = Round Toward -Infinity(1:w549) -> (0:w545:dbl)
                  n104 = Multiply(x=w545, y=w544) -> (x*y=w543:dbl)
                  n105 = Add(x=w543, y=w537) -> (x+y=w542:dbl)
                  n106 = Increment(x=w542) -> (x+1=w541:dbl)
                  n107 = Subtract(x=w541, y=w538) -> (x-y=w546:dbl)
                }
              }
              n108 = Subtract(x=w519, y=w520) -> (x-y=w514:dbl)
              n109 = Decrement(x=w514) -> (x-1=w513:dbl)
              n110 = Max & Min(x=0, y=w513) -> (max(x,y)=w512:dbl)  [unwired: 1 out]
              n111 = Divide(x=w512, y=w519) -> (x/y=w526:dbl)
              n112 = Greater Than 0?(x=w512) -> (x > 0?=w516:bool)
              n113 = Select(t=u32 16711680, s=w516, f=u32 0) -> (s? t:f=w527:u32)
              n114 = Multiply(x=w526, y=100.0) -> (x*y=w524:dbl)
              n115 = Format Into String(format string="%d / %.1f%%" ("Format-String"), w512, w524) -> (resulting string=→"COM-Fehlerrate":string)  [unwired: 2 in, 1 out]
              n116 = property on="COM-Fehlerrate" class="Str"("Text.TextColor"=w527) -> ()  [unwired: 2 in, 2 out]
            }
          }
          n117 = case "Case-Struktur" shown="True" w440 {
            tunnel: w499 -> [w703 w714]
            tunnel: w498 -> [w702 w713]
            tunnel: [w703 w712] -> w497
            tunnel: [w702 w711] -> w496
            tunnel: w457 -> [_ w705]
            tunnel: w432 -> [w701 _]
            tunnel: [w701 w704] -> w462
            tunnel: w459 -> [_ w710]
            tunnel: "Rollenumfang [m]" -> [_ w709]
            frame False {
            }
            frame True {
              w721 = 60.0 ("y")
              n118 = Reciprocal "Abtastzeit [s]"(x=w705) -> (1/x=w704:dbl)
              n119 = Divide "R [1/s]"(x=w713, y="Rollengeber [Inkr/U]") -> (x/y=w720:dbl)
              n120 = Divide(x=w714, y="Zündung [Imp/U]") -> (x/y=w717:dbl)
              n121 = Multiply "nZ gemessen [1/min]"(x=w717, y=w721) -> (x*y=w712:dbl)
              n122 = Multiply "nR [1/min]"(x=w721, y=w720) -> (x*y=w711:dbl)
              n123 = Multiply "nZ berechnet [1/min]"(x=w711, y=w710) -> (x*y=w719:dbl)
              n124 = Multiply "[m/min]"(x=w711, y=w709) -> (x*y=w715:dbl)
              n125 = Multiply "[km/h]"(x=w715, y=0.06) -> (x*y=→"Hinterrad\n[km/h]":dbl)
              n126 = Bundle(w712, w719) -> (→"Welle\n[1/min]":cluster{dbl, dbl})  [unwired: 1 in]
            }
          }
          n127 = case shown="True" w440 {
            tunnel: w497 -> [_ w629]
            tunnel: w496 -> [_ w628]
            tunnel: "Rollenumfang [m]" -> [_ w632]
            tunnel: [w561 w602] -> w427
            tunnel: w459 -> [w550 w602]
            tunnel: w472 -> [w562 w636]
            tunnel: w495 -> [w563 w635]
            tunnel: [w562 w594] -> w430
            tunnel: [w563 w634] -> w458
            tunnel: w439 -> [_ w631]
            tunnel: w444 -> [_ w630]
            tunnel: [w560 w573] -> w492
            tunnel: [w559 w574] -> w491
            tunnel: w490 -> [w560 w627]
            tunnel: w489 -> [w559 _]
            tunnel: w443 -> [_ w583]
            tunnel: [w558 w608] -> w478
            tunnel: w488 -> [w558 _]
            tunnel: [w557 w571] -> w482
            tunnel: w486 -> [w557 _]
            tunnel: [w556 w609] -> w481
            tunnel: w487 -> [w556 _]
            tunnel: [w555 w621] -> w480
            tunnel: w485 -> [w555 _]
            tunnel: [w554 w620] -> w479
            tunnel: w484 -> [w554 _]
            tunnel: w445 -> [_ w613]
            tunnel: w475 -> [w553 w607]
            tunnel: "n vom Gas [1/min]" -> [_ w596]
            tunnel: [w553 w606] -> w473
            tunnel: w472 -> [_ w605]
            tunnel: w436 -> [w552 w601]
            tunnel: [w552 w600] -> w469
            tunnel: w462 -> [_ w599]
            tunnel: [w551 w572] -> w435
            tunnel: w461 -> [w551 w598]
            tunnel: w434 -> [_ w581]
            tunnel: w433 -> [_ w580]
            frame False {
              n128 = case shown="False" w562 {
                tunnel: w563 -> [w567 _]
                tunnel: [w566 w568] -> w561
                tunnel: w550 -> [_ w568]
                frame False {
                  n129 = call <vilib>:"Measures of Mean.vi"("percent (trim)"=20.0, "type"=3, "x array"=w567) -> ("mean value"=w566:dbl)  [unwired: 7 in, 1 out]
                }
                frame True {
                }
              }
            }
            frame True {
              w616 = 0.00135962  # [W] in [PS]
              w623 = 0.10471975511965978  # 2*Pi/60
              n130 = local read "Differenzenquotient"() -> (w579:u8)
              n131 = Build Array (concatenate) "akt. dT in Array einfügen"(w598, w599) -> (w572:dbl[])
              n132 = Build Array (concatenate) "akt. Rollendrehzahl\nin Array einfügen"(w627, w628) -> (w573:dbl[])
              n133 = local read "Übersetzung ermitteln aus"() -> (w569:T2)
              n134 = Multiply(x=2, y=w579) -> (x*y=w577:i32)
              n135 = Increment(x=w577) -> (x+1=w575:i32)
              n136 = Index Array(array=w572, index=1 ("Index")) -> (element=w586:dbl)
              n137 = Index Array(array=w573, index=1 ("Index")) -> (element=w592:dbl)
              n138 = case shown="\"Getriebe & Reifen\"" w569 {
                tunnel: w629 -> [_ _ w700]
                tunnel: w628 -> [_ _ w699]
                tunnel: [w695 "nKuWe/nRolle" w698] -> w633
                tunnel: w632 -> [w696 _ _]
                frame "Getriebe & Reifen" {
                  n139 = Divide(x=w696, y="Reifenumfang [m]") -> (x/y=w694:dbl)
                  n140 = Multiply(x=w694, y="Getriebe [1:]") -> (x*y=w695:dbl)
                }
                frame "nKuWe / nRolle" {
                }
                frame "Zündsignal" {
                  n141 = Divide(x=w700, y=w699) -> (x/y=w698:dbl)
                }
              }
              n142 = Initialize Array(w586, w575) -> (w584:dbl[])
              n143 = Initialize Array(w592, w583) -> (w591:dbl[])
              n144 = Insert Into Array(array=w573, index=0 ("Index"), new element=w591) -> (w589:dbl[])
              n145 = Insert Into Array(array=w572, index=0 ("Index"), new element=w584) -> (w582:dbl[])
              n146 = call-poly <vilib>:"IIR Filter.vi"("Forward Coefficients"=w630, "Reverse Coefficients"=w631, "X"=w589) -> ("Filtered X"=w588:dbl[])  [unwired: 1 in, 1 out]
              n147 = call-poly <vilib>:"IIR Filter.vi"("Forward Coefficients"=w580, "Reverse Coefficients"=w581, "X"=w582) -> ("Filtered X"=w576:dbl[])  [unwired: 1 in, 1 out]
              n148 = Array Subset "Rolle gefiltert [1/min]"(array=w588, index=w583) -> (w574:dbl[])  [unwired: 1 in]
              n149 = Array Subset "dT gefiltert [s]"(array=w576, index=w575) -> (w570:dbl[])  [unwired: 1 in]
              n150 = case shown="False" w636 {
                selector: w636 -> [_ w691]
                tunnel: w633 -> [w679 _]
                tunnel: w635 -> [w681 w690]
                tunnel: [w676 w691] -> w626
                tunnel: [w680 w690] -> w634
                tunnel: w601 -> [w678 w689]
                tunnel: [w676 w689] -> w600
                tunnel: w569 -> [w675 _]
                frame False {
                  n151 = Build Array (concatenate)(w681, w679) -> (w680:dbl[])
                  n152 = case shown="\"Zündsignal\"" w675 {
                    tunnel: ["Dauer [s]" 0.0 ("Dauer [s]") 0.0] -> w677
                    frame "Zündsignal" {
                      n153 = property on="Untersetzung\nermittelt" class="Bool. (strikt)"("Blinking"=TRUE ("Blinkend"), "BoolText.Text"="Ermittle Übersetzung" ("Boolescher Text.Text")) -> ()  [unwired: 2 in, 2 out]
                    }
                    frame "Getriebe & Reifen", Default {
                    }
                    frame "nKuWe / nRolle" {
                    }
                  }
                  n154 = call "Verstrichene Zeit"("Time Target (s)"=w677, "Reset"=w678) -> ("Time has Elapsed"=w676:bool)  [unwired: 10 in, 7 out]
                  n155 = case shown="True" w676 {
                    frame False {
                    }
                    frame True {
                      n156 = property on="Untersetzung\nermittelt" class="Bool. (strikt)"("Blinking"=FALSE ("Blinkend"), "BoolText.Text"="Go" ("Boolescher Text.Text")) -> ()  [unwired: 2 in, 2 out]
                    }
                  }
                  "Untersetzung-Graph" <- w679
                }
                frame True {
                }
              }
              n157 = Array Size "Array-Größe"(array=w574) -> (size(s)=w624:i32)
              n158 = Square(x=w602) -> (x^2=w622:dbl)
              n159 = Multiply(x=w574, y=w602) -> (x*y=w608:dbl[])
              n160 = Multiply(x=w608, y=w623) -> (x*y=w571:dbl[])
              n161 = Greater?(x=w624, y=w583) -> (0:w625:bool)
              n162 = Divide(x="Rollenträgheit [kgm²]", y=w622) -> (x/y=w614:dbl)
              n163 = Multiply(x=w614, y=w613) -> (x*y=w612:dbl)
              n164 = And(x=w626, y=w625) -> (x .and. y?=w594:bool)
              n165 = Array Size "Array-Größe"(array=w571) -> (size(s)=w611:i32)
              n166 = Decrement(x=w611) -> (x-1=w610:i32)
              n167 = Select(t=w596, s=w594, f=1000000.0) -> (s? t:f=w597:dbl)
              n168 = Initialize Array(0.0 ("y"), 0) -> (w617:dbl[])
              n169 = for {
                N: w611 -> [_]
                tunnel: "Differenzenquotient" -> [w651]
                tunnel: w571 -> [w659]
                tunnel: w610 -> [w650]
                shift-right: [w656] -> w609
                shift-left: w617 -> [w657]
                tunnel: w608 -> [w654] mode=indexing
                tunnel: w607 -> [w643]
                tunnel: w597 -> [w653]
                tunnel: [w644] -> w606
                tunnel: w605 -> [w641]
                tunnel: w570 -> [w638] mode=indexing
                i -> [w639]
                stop <- w642 stop-if-true
                n170 = Subtract(x=w650, y=w651) -> (x-y=w652:i32)
                n171 = Add(x=w639, y=w651) -> (x+y=w666:i32)
                n172 = Subtract(x=w639, y=w651) -> (x-y=w672:i32)
                n173 = Greater Or Equal?(x=w639, y=w651) -> (x >= y?=w647:bool)
                n174 = Greater?(x=w654, y=w653) -> (0:w655:bool)
                n175 = Max & Min(x=w650, y=w666) -> (min(x,y)=w667:i32)  [unwired: 1 out]
                n176 = Max & Min(x=w672, y=0) -> (max(x,y)=w670:i32)  [unwired: 1 out]
                n177 = Subtract(x=w667, y=w639) -> (x-y=w668:i32)
                n178 = Subtract(x=w639, y=w670) -> (x-y=w669:i32)
                n179 = Less Or Equal?(x=w639, y=w652) -> (x <= y?=w648:bool)
                n180 = Max & Min(x=w669, y=w668) -> (min(x,y)=w660:i32)  [unwired: 1 out]
                n181 = Multiply(x=w638, y=2.0) -> (x*y=w640:dbl)
                n182 = Add(x=w639, y=w660) -> (x+y=w665:i32)
                n183 = Subtract(x=w639, y=w660) -> (x-y=w664:i32)
                n184 = Multiply(x=w660, y=w640) -> (x*y=w658:dbl)
                n185 = Index Array(array=w659, index=w665) -> (element=w662:dbl)
                n186 = Index Array(array=w659, index=w664) -> (element=w663:dbl)
                n187 = Subtract(x=w662, y=w663) -> (x-y=w661:dbl)
                n188 = Divide(x=w661, y=w658) -> (x/y=w649:dbl)
                n189 = Less Than 0?(x=w649) -> (x < 0?=w646:bool)
                n190 = Less Or Equal To 0?(x=w643) -> (x <= 0?=w645:bool)
                n191 = Build Array (concatenate)(w657, w649) -> (w656:dbl[])
                n192 = Compound Arithmetic op=AND(w646, w655, w645, w647, w648, w641) -> (w642:bool)
                n193 = case shown="False" w642 {
                  tunnel: w639 -> [_ w674]
                  tunnel: [w673 w674] -> w644
                  tunnel: w643 -> [w673 _]
                  frame False {
                  }
                  frame True {
                  }
                }
              }
              n194 = Multiply(x=w609, y=w612) -> (x*y=w621:dbl[])
              n195 = Multiply(x=w571, y=w621) -> (x*y=w615:dbl[])
              n196 = Multiply(x=w616, y=w615) -> (x*y=w620:dbl[])
            }
          }
          "Untersetzung\nermittelt" <- w430
          n197 = local read "Übersetzung ermitteln aus"() -> (w431:T2)
          n198 = Greater Than 0?(x=w473) -> (x > 0?=w474:bool)
          n199 = Select(t=w427, s=w430, f=0.0) -> (s? t:f=→"Untersetzung":dbl)
          n200 = Equal To 0? "aus Zündsignal?"(x=w431) -> (x = 0?=w429:bool)
          n201 = local read "Start"() -> (w442:bool)
          n202 = And(x=w430, y=w429) -> (x .and. y?=w428:bool)
          n203 = case shown="True" w428 {
            tunnel: w427 -> [_ w505]
            frame False {
            }
            frame True {
              n204 = local write "nKuWe/nRolle"(w505) -> ()
            }
          }
          n205 = Not(x=w442) -> (.not. x?=w441:bool)
          n206 = Or(x=w474, y=w441) -> (x .or. y?=w477:bool)
        }
        n207 = VISA Clear(VISA resource name=w10, error in (no error)=w9) -> (VISA resource name out=w7:refnum<visa-resource-name>, error out=w11:errorcluster)
        n208 = VISA Close(VISA resource name=w7, error in (no error)=w11) -> ()  [unwired: 1 out]
        n209 = case shown="True" w38 {
          tunnel: w36 -> [_ w403]
          tunnel: w35 -> [_ w408]
          tunnel: w34 -> [_ w407]
          tunnel: w33 -> [_ w379]
          tunnel: w6 -> [_ w404]
          tunnel: w32 -> [_ w402]
          tunnel: w31 -> [_ w396]
          tunnel: w26 -> [_ w382]
          tunnel: ["" w381] -> w27
          tunnel: w28 -> [_ w380]
          tunnel: ["" w378] -> _
          tunnel: [w362 w366] -> _
          frame False {
            w363 = 0.0
            n210 = Initialize Array(w363, w363) -> (w362:dbl[])
          }
          frame True {
            w377 = 0
            n211 = Array Subset "P"(array=w407, length=w379) -> (w399:dbl[])  [unwired: 1 in]
            n212 = Array Subset "M"(array=w408, length=w379) -> (w400:dbl[])  [unwired: 1 in]
            n213 = Array Subset "alpha"(array=w404, length=w379) -> (w405:dbl[])  [unwired: 1 in]
            n214 = Array Subset "n"(array=w403, length=w379) -> (w401:dbl[])  [unwired: 1 in]
            n215 = property on="Pmax" class="Str"("Text.FontSize"=48) -> ()  [unwired: 2 in, 2 out]
            n216 = property on="Ergebnis" class="Str"("Text.FontSize"=18) -> ()  [unwired: 2 in, 2 out]
            n217 = Array Size(array=w405) -> (size(s)=w406:i32)
            n218 = for {
              N: w406 -> [w426]
              tunnel: w404 -> [w423]
              tunnel: w403 -> [w420]
              tunnel: w402 -> [w417]
              tunnel: [w415] -> w376
              i -> [w421]
              stop <- w416 stop-if-true
              n219 = Decrement(x=w426) -> (x-1=w425:i32)
              n220 = Subtract(x=w425, y=w421) -> (x-y=w415:i32)
              n221 = Index Array(array=w423, index=w415) -> (element=w424:dbl)
              n222 = Index Array(array=w420, index=w415) -> (element=w419:dbl)
              n223 = Less?(x=w419, y=w417) -> (x < y?=w418:bool)
              n224 = Less Or Equal To 0?(x=w424) -> (x <= 0?=w422:bool)
              n225 = And(x=w422, y=w418) -> (x .and. y?=w416:bool)
            }
            n226 = Increment(x=w376) -> (x+1=w375:i32)
            n227 = Array Subset "P"(array=w399, index=w375) -> (w367:dbl[])  [unwired: 1 in]
            n228 = Array Subset "M"(array=w400, index=w375) -> (w366:dbl[])  [unwired: 1 in]
            n229 = Array Subset "n"(array=w401, index=w375) -> (w372:dbl[])  [unwired: 1 in]
            n230 = Bundle(w372, w367) -> (w371:cluster{dbl[], dbl[]})  [unwired: 1 in]
            n231 = Bundle(w372, w366) -> (w370:cluster{dbl[], dbl[]})  [unwired: 1 in]
            n232 = Array Max & Min "nmax [1/min]"(array=w372) -> (max value=w398:dbl)  [unwired: 3 out]
            n233 = Divide(x=w398, y=w380) -> (x/y=w397:dbl)
            n234 = Compound Arithmetic op=MULTIPLY "vmax"(w397, w396, 0.06) -> (w388:dbl)
            n235 = Array Max & Min "Mmax"(array=w366) -> (max value=w373:dbl, max index (indices)=w369:i32)  [unwired: 2 out]
            n236 = Multiply(x=w373, y=1.8) -> (x*y=w409:dbl)
            n237 = Index Array "n(Mmax)"(array=w372, index=w369) -> (element=w389:dbl)
            n238 = Array Max & Min "Pmax"(array=w367) -> (max value=w374:dbl, max index (indices)=w368:i32)  [unwired: 2 out]
            n239 = Build Array(w371, w370) -> (→"XY-Graph":cluster{dbl[], dbl[]}[])
            n240 = local read "Luftfeuchtigkeit [%]"() -> (w392:dbl)
            n241 = local read "Lufttemperatur [°C]"() -> (w391:dbl)
            n242 = local read "Luftdruck [mbar]"() -> (w393:dbl)
            n243 = Multiply(x=w374, y=1.2) -> (x*y=w410:dbl)
            n244 = property on="XY-Graph" class="XYGraph (strikt)"("ActYScl"=1, "YScale.Maximum"=w409, "YScale.Minimum"=w377) -> ()  [unwired: 2 in, 2 out]
            n245 = property on="XY-Graph" class="XYGraph (strikt)"("ActYScl"=w377, "YScale.Maximum"=w410, "YScale.Minimum"=w377) -> ()  [unwired: 2 in, 2 out]
            n246 = Index Array "n(Pmax)"(array=w372, index=w368) -> (element=w394:dbl)
            n247 = Format Into String(format string="%.1f PS" ("Format-String"), w374) -> (resulting string=→"Pmax":string)  [unwired: 2 in, 1 out]
            n248 = Format Date/Time String(time format string (%c)="%x %H:%M ") -> (date/time string=w381:string)  [unwired: 2 in]
            n249 = Format Into String(format string="%.1f PS bei %d 1/min   |   %.1f Nm bei %d 1/min   |   vmax: %d km/h\\nDIN 70020 k =%.3f (%d \\B0C, %d %%, %d mbar)\\n%s" ("Format-String"), w374, w394, w373, w389, w388, w382, w391, w392, w393, w381) -> (resulting string=w378:string)  [unwired: 2 in, 1 out]
            "Ergebnis" <- w378
          }
        }
        n250 = flat-sequence {
          tunnel: w20 -> [w325]
          tunnel: w22 -> [w326]
          tunnel: w25 -> [w327]
          tunnel: w26 -> [w328]
          tunnel: w27 -> [w329]
          tunnel: w28 -> [w330]
          tunnel: w29 -> [w331]
          tunnel: w30 -> [w332]
          tunnel: [w332] -> w124
          tunnel: [w331] -> w123
          tunnel: [w330] -> w122
          tunnel: [w329] -> w121
          tunnel: [w328] -> w120
          tunnel: [w327] -> w119
          tunnel: [w326] -> w118
          tunnel: [w325] -> w117
          tunnel: [w321] -> w8
          tunnel: w7 -> [w321]
          tunnel: w124 -> [w361]
          tunnel: w123 -> [w360]
          tunnel: w122 -> [w359]
          tunnel: w121 -> [w358]
          tunnel: w120 -> [w357]
          tunnel: w119 -> [w356]
          tunnel: w118 -> [w355]
          tunnel: w117 -> [w354]
          tunnel: w8 -> [w336]
          frame #0 {
            w323 = FALSE ("Start [F1]")
            w324 = 0  # Aktivieren
            n251 = local write "Start"(w323) -> ()
            n252 = property on="Speichern" class="Bool. (strikt)"("DisabledEnum"=w324) -> ()  [unwired: 2 in, 2 out]
            n253 = property on="Übersetzung ermitteln aus" class="Enum (strikt)"("DisabledEnum"=w324) -> ()  [unwired: 2 in, 2 out]
            n254 = property on="Konfiguration:" class="Bool. (strikt)"("DisabledEnum"=w324) -> ()  [unwired: 2 in, 2 out]
            n255 = property on="Ende" class="Bool. (strikt)"("DisabledEnum"=w324) -> ()  [unwired: 2 in, 2 out]
            n256 = property on="Drucken" class="Bool. (strikt)"("DisabledEnum"=w324) -> ()  [unwired: 2 in, 2 out]
            n257 = property on="Untersetzung\nermittelt" class="Bool. (strikt)"("BoolText.Text"="GO" ("Boolescher Text.Text"), "Blinking"=w323) -> ()  [unwired: 2 in, 2 out]
            n258 = local write "Untersetzung\nermittelt"(w323) -> ()
          }
          frame #1 {
            w333 = dbl[] []
            w339 = 0.0
            n259 = local read "Übersetzung ermitteln aus"() -> (w342:T2)
            n260 = local read "Rollenträgheit [kgm²]"() -> (w351:dbl)
            n261 = local read "Gleitender Mittelwert"() -> (w347:u8)
            n262 = local read "Messung Klimadaten"() -> (w338:bool)
            n263 = local read "Rollengeber [Inkr/U]"() -> (w352:u16)
            n264 = local read "Differenzenquotient"() -> (w346:u8)
            n265 = local read "Lufttemperatur [°C]"() -> (w345:dbl)
            n266 = local read "Luftfeuchtigkeit [%]"() -> (w344:dbl)
            n267 = local read "Reifenumfang [m]"() -> (w348:dbl)
            n268 = local read "n vom Gas [1/min]"() -> (w340:dbl)
            n269 = local read "Zündung [Imp/U]"() -> (w350:dbl)
            n270 = local read "Luftdruck [mbar]"() -> (w343:dbl)
            n271 = local read "nKuWe/nRolle"() -> (w335:dbl)
            n272 = local read "Getriebe [1:]"() -> (w349:dbl)
            n273 = local read "Dauer [s]"() -> (w341:dbl)
            n274 = Bundle("Fahrzeugdaten"="Fahrzeugdaten", "date/time string"=w358, "Rollengeber [Inkr/U]"=w352, "Rollenumfang [m]"=w356, "Rollenträgheit [kgm²]"=w351, "Zündung [Imp/U]"=w350, "Getriebe [1:]"=w349, "Reifenumfang [m]"=w348, "mean value"=w359, "Gleitender Mittelwert"=w347, "Differenzenquotient"=w346, 0, w361, "element"=w357, "Lufttemperatur [°C]"=w345, "Luftfeuchtigkeit [%]"=w344, "Luftdruck [mbar]"=w343, w360, w333, w333, w333, "Übersetzung ermitteln aus"=w342, "Dauer [s]"=w341, w339, w339, "n vom Gas [1/min]"=w340, w355, w354, "Messung Klimadaten"=w338, "VISA resource name out"=w336, "nKuWe/nRolle"=w335) -> (→"Datenspeicher":T5)  [unwired: 1 in]
          }
        }
      }
    }
    n275 = local read "Ende"() -> (w1:bool)
  }
  n276 = flat-sequence {
    frame #0 {
      n277 = call <vilib>:"Application Directory.vi"() -> ("Application Directory"=w817:path)
      n278 = Build Path(base path=w817, name or relative path="Konfig.xml") -> (appended path=w815:path)
      n279 = call-poly <vilib>:"Read From XML File.vi"("XML File Path"=w815) -> ("error out"=w797:errorcluster, "XML Elements"=w819:string)  [unwired: 8 in, 1 out]
      n280 = property on="Datenspeicher" class="Cluster (strikt)"() -> ("Value"=w818:T3)  [unwired: 2 in, 2 out]
      n281 = case shown="Kein Fehler" w797 {
        tunnel: w819 -> [w822 _]
        tunnel: w818 -> [w821 _]
        tunnel: [w820 T6 {"Fahrzeugdaten"="", "date/time string"="05.02.2017 22:14 ", "Rolle [Inkr/U]"=10, "Rollenumfang [m]"=0.613, "Rollenträgheit [kgm²]"=0.402, "Zündung [Imp/U]"=5.0, "Getriebe [1:]"=5.343, "Reifenumfang [m] "=1.222, "element"=2.0, "Gl. Mittelwert"=35, "Differenzenquotient"=12, "Polynom"=15, "element"=0.01639344262295082, "element"=1.0177230216140456, "Lufttemperatur [°C]"=23.3, "Luftfeuchtigkeit [%]"=43.8, "Luftdruck [mbar]"=1013.45, array[1238 elements], array[1224 elements], "Best Polynomial Fit"=array[1224 elements], array[1224 elements], "Übersetzung ermitteln aus"=0, "[s]"=5.0, "nmin [1/min]"=0.0, "nmax [1/min]"=0.0, "n vom Gas [1/min]"=5000.0, array[1238 elements], array[1238 elements], "Boolesch"=TRUE, "Serielle Schnittstelle"="", 10.0} ("Datenspeicher")] -> w798
        frame No Error {
          n282 = Unflatten From XML(xml string=w822, type=w821) -> (value=w820:T3)  [unwired: 1 in, 1 out]
        }
        frame Error {
        }
      }
      n283 = property on="Datenspeicher" class="Cluster (strikt)"("Value"=w798) -> ()  [unwired: 2 in, 2 out]
      n284 = Unbundle(w798) -> ("Fahrzeugdaten"=w814:string, "Rolle [Inkr/U]"=w813:u16, "Rollenumfang [m]"=w812:dbl, "Rollenträgheit [kgm²]"=w811:dbl, "Zündung [Imp/U]"=w810:dbl, "Getriebe [1:]"=w809:dbl, "Reifenumfang [m]"=w808:dbl, "element"=w796:dbl, "Gl. Mittelwert"=w807:u8, "Differenzenquotient"=w806:u8, "Lufttemperatur [°C]"=w805:dbl, "Luftfeuchtigkeit [%]"=w804:dbl, "Luftdruck [mbar]"=w803:dbl, "Übersetzung ermitteln aus"=w800:u8, "[s]"=w802:dbl, "n vom Gas [1/min]"=w801:dbl, "Boolesch"=w799:bool, "Serielle Schnittstelle"=w795:refnum<visa-resource-name>, "nKuWe/nRolle"=w794:dbl)  [unwired: 12 out]
      n285 = property on="Dauer [s]" class="DigWert (strikt)"("Value"=w802) -> ()  [unwired: 2 in, 2 out]
      n286 = property on="Fahrzeugdaten" class="Str"("Value"=w814) -> ()  [unwired: 2 in, 2 out]
      n287 = property on="Rollengeber [Inkr/U]" class="DigWert (strikt)"("Value"=w813) -> ()  [unwired: 2 in, 2 out]
      n288 = property on="Rollenumfang [m]" class="DigWert (strikt)"("Value"=w812) -> ()  [unwired: 2 in, 2 out]
      n289 = property on="Rollenträgheit [kgm²]" class="DigWert (strikt)"("Value"=w811) -> ()  [unwired: 2 in, 2 out]
      n290 = property on="Zündung [Imp/U]" class="DigWert (strikt)"("Value"=w810) -> ()  [unwired: 2 in, 2 out]
      n291 = property on="Getriebe [1:]" class="DigWert (strikt)"("Value"=w809) -> ()  [unwired: 2 in, 2 out]
      n292 = property on="Reifenumfang [m]" class="DigWert (strikt)"("Value"=w808) -> ()  [unwired: 2 in, 2 out]
      n293 = property on="nKuWe/nRolle" class="DigWert (strikt)"("Value"=w796) -> ()  [unwired: 2 in, 2 out]
      n294 = property on="Gleitender Mittelwert" class="DigWert (strikt)"("Value"=w807) -> ()  [unwired: 2 in, 2 out]
      n295 = property on="Differenzenquotient" class="DigWert (strikt)"("Value"=w806) -> ()  [unwired: 2 in, 2 out]
      n296 = property on="Lufttemperatur [°C]" class="DigWert (strikt)"("Value"=w805) -> ()  [unwired: 2 in, 2 out]
      n297 = property on="Luftfeuchtigkeit [%]" class="DigWert (strikt)"("Value"=w804) -> ()  [unwired: 2 in, 2 out]
      n298 = property on="Luftdruck [mbar]" class="DigWert (strikt)"("Value"=w803) -> ()  [unwired: 2 in, 2 out]
      n299 = property on="Übersetzung ermitteln aus" class="Enum (strikt)"("Val(Sgnl)"=w800) -> ()  [unwired: 2 in, 2 out]
      n300 = property on="n vom Gas [1/min]" class="DigWert (strikt)"("Value"=w801) -> ()  [unwired: 2 in, 2 out]
      n301 = property on="Messung Klimadaten" class="Bool. (strikt)"("Val(Sgnl)"=w799) -> ()  [unwired: 2 in, 2 out]
      n302 = local write "Serielle Schnittstelle"(w795) -> ()
      n303 = property on="nKuWe/nRolle" class="DigWert (strikt)"("Value"=w794) -> ()  [unwired: 2 in, 2 out]
    }
    frame #1 {
      w830 = 2  # Deaktivieren
      w832 = 0.0  # Graphen löschen
      n304 = local read "Serielle Schnittstelle"() -> (w828:refnum<visa-resource-name>)
      n305 = property on="Frontpanel-Position" class="Bereich"("Origin"=T7 {"Horizontal"=8, "Vertical"=6}) -> ()  [unwired: 2 in, 2 out]
      n306 = property on="Füllstand Lesepuffer" class="Schieber (strikt)"("Scale.Maximum"=100) -> ()  [unwired: 2 in, 2 out]
      n307 = property on="Drucken" class="Bool. (strikt)"("DisabledEnum"=w830) -> ()  [unwired: 2 in, 2 out]
      n308 = property on="Speichern" class="Bool. (strikt)"("DisabledEnum"=w830) -> ()  [unwired: 2 in, 2 out]
      n309 = Build Array(w832) -> (w831:dbl[])
      n310 = VISA Clear(VISA resource name=w828) -> (VISA resource name out=w827:refnum<visa-resource-name>, error out=w826:errorcluster)  [unwired: 1 in]
      n311 = property on="Untersetzung-Graph" class="SVDiagr (strikt)"("History Data"=w831) -> ()  [unwired: 2 in, 2 out]
      n312 = VISA Close(VISA resource name=w827, error in (no error)=w826) -> (error out=w825:errorcluster)
      n313 = case shown="Kein Fehler" w825 {
        tunnel: [T4."Enabled" ("Deaktiviert") T4."Disabled and Grayed Out" ("Deaktiviert")] -> w824
        frame No Error {
        }
        frame Error {
        }
      }
      n314 = property on="Start" class="Bool. (strikt)"("DisabledEnum"=w824) -> ()  [unwired: 2 in, 2 out]
    }
  }
  n315 = while {
    stop <- w836 stop-if-true
    n316 = event shown="[2] \"Speichern\": Wertänderung" {
      selector: _ -> [_ _ _ _ _ _ _ _]
      dyn-events: _ -> [_ _ _ _ _ _ _ _]
      timeout: _ -> [_ _ _ _ _ _ _ _]
      tunnel: [_ _ _ TRUE _ _ _ _] -> w836
      event "Konfiguration:": Value Change {
        n317 = event-data() -> ("OldVal"=w838:bool)  [unwired: 1 in, 5 out]
        n318 = flat-sequence {
          tunnel: [w842] -> w839
          tunnel: w838 -> [w842]
          tunnel: w839 -> [w868]
          frame #0 {
            n319 = call-poly <vilib>:"Read From XML File.vi"() -> ("error out"=w840:errorcluster, "XML Elements"=w843:string)  [unwired: 9 in, 1 out]
            n320 = property on="Datenspeicher" class="Cluster (strikt)"() -> ("Value"=w841:T3)  [unwired: 2 in, 2 out]
            n321 = case shown="Kein Fehler" w840 {
              selector: w840 -> [_ w867]
              tunnel: w843 -> [w847 _]
              tunnel: w841 -> [w846 _]
              frame No Error {
                n322 = Unflatten From XML(xml string=w847, type=w846) -> (value=w845:T3, error out=w844:errorcluster)  [unwired: 1 in]
                n323 = case shown="Kein Fehler" w844 {
                  tunnel: w845 -> [w865 _]
                  frame No Error {
                    n324 = Unbundle(w865) -> ("Fahrzeugdaten"=w864:string, "Rolle [Inkr/U]"=w863:u16, "Rollenumfang [m]"=w862:dbl, "Rollenträgheit [kgm²]"=w861:dbl, "Zündung [Imp/U]"=w860:dbl, "Getriebe [1:]"=w859:dbl, "Reifenumfang [m]"=w858:dbl, "Gl. Mittelwert"=w857:u8, "Differenzenquotient"=w856:u8, "Lufttemperatur [°C]"=w855:dbl, "Luftfeuchtigkeit [%]"=w854:dbl, "Luftdruck [mbar]"=w853:dbl, "Übersetzung ermitteln aus"=w850:u8, "[s]"=w852:dbl, "n vom Gas [1/min]"=w851:dbl, "Boolesch"=w849:bool, "nKuWe/nRolle"=w848:dbl)  [unwired: 14 out]
                    n325 = property on="Dauer [s]" class="DigWert (strikt)"("Value"=w852) -> ()  [unwired: 2 in, 2 out]
                    n326 = property on="Fahrzeugdaten" class="Str"("Value"=w864) -> ()  [unwired: 2 in, 2 out]
                    n327 = property on="Rollengeber [Inkr/U]" class="DigWert (strikt)"("Value"=w863) -> ()  [unwired: 2 in, 2 out]
                    n328 = property on="Rollenumfang [m]" class="DigWert (strikt)"("Value"=w862) -> ()  [unwired: 2 in, 2 out]
                    n329 = property on="Rollenträgheit [kgm²]" class="DigWert (strikt)"("Value"=w861) -> ()  [unwired: 2 in, 2 out]
                    n330 = property on="Zündung [Imp/U]" class="DigWert (strikt)"("Value"=w860) -> ()  [unwired: 2 in, 2 out]
                    n331 = property on="Getriebe [1:]" class="DigWert (strikt)"("Value"=w859) -> ()  [unwired: 2 in, 2 out]
                    n332 = property on="Reifenumfang [m]" class="DigWert (strikt)"("Value"=w858) -> ()  [unwired: 2 in, 2 out]
                    n333 = property on="Gleitender Mittelwert" class="DigWert (strikt)"("Value"=w857) -> ()  [unwired: 2 in, 2 out]
                    n334 = property on="Differenzenquotient" class="DigWert (strikt)"("Value"=w856) -> ()  [unwired: 2 in, 2 out]
                    n335 = property on="Lufttemperatur [°C]" class="DigWert (strikt)"("Value"=w855) -> ()  [unwired: 2 in, 2 out]
                    n336 = property on="Luftfeuchtigkeit [%]" class="DigWert (strikt)"("Value"=w854) -> ()  [unwired: 2 in, 2 out]
                    n337 = property on="Luftdruck [mbar]" class="DigWert (strikt)"("Value"=w853) -> ()  [unwired: 2 in, 2 out]
                    n338 = property on="Übersetzung ermitteln aus" class="Enum (strikt)"("Val(Sgnl)"=w850) -> ()  [unwired: 2 in, 2 out]
                    n339 = property on="n vom Gas [1/min]" class="DigWert (strikt)"("Value"=w851) -> ()  [unwired: 2 in, 2 out]
                    n340 = property on="Messung Klimadaten" class="Bool. (strikt)"("Val(Sgnl)"=w849) -> ()  [unwired: 2 in, 2 out]
                    n341 = property on="nKuWe/nRolle" class="DigWert (strikt)"("Value"=w848) -> ()  [unwired: 2 in, 2 out]
                  }
                  frame Error {
                    n342 = One Button Dialog(message="Dateiversion nicht kompatibel" ("Nachricht")) -> ()  [unwired: 1 in, 1 out]
                  }
                }
              }
              frame Error {
                n343 = call <vilib>:"Clear Errors.vi"("error in (no error)"=w867) -> ()  [unwired: 5 in, 2 out]
              }
            }
          }
          frame #1 {
            n344 = property on="Konfiguration:" class="Bool. (strikt)"("Value"=w868) -> ()  [unwired: 2 in, 2 out]
          }
        }
      }
      event "Drucken": Value Change {
        n345 = event-data() -> ("OldVal"=w869:bool)  [unwired: 1 in, 5 out]
        n346 = flat-sequence {
          tunnel: [w874] -> w870
          tunnel: w869 -> [w874]
          tunnel: w870 -> [w875]
          frame #0 {
            n347 = control-ref of="Fahrzeugdaten"() -> (w872:refnum<vi>)
            n348 = control-ref of="XY-Graph"() -> (w873:refnum<vi>)
            n349 = control-ref of="Ergebnis"() -> (w871:refnum<vi>)
            n350 = call "printgraph_V0.01.vi"("reference 2"=w871, "Fahrzeugdaten"=w872, "XYGraph (Eingang)"=w873) -> ()  [unwired: 9 in]
          }
          frame #1 {
            n351 = property on="Drucken" class="Bool. (strikt)"("Value"=w875) -> ()  [unwired: 2 in, 2 out]
          }
        }
      }
      event "Speichern": Value Change {
        n352 = event-data() -> ("OldVal"=w877:bool)  [unwired: 1 in, 5 out]
        n353 = control-ref of="Datenspeicher"() -> (w876:refnum<vi>)
        n354 = local write "Speichern"(w877) -> ()
        n355 = call "savecluster_V0.01.vi"("Datenspeicher 3"=w876) -> ()  [unwired: 2 in]
      }
      event "Ende": Value Change {
        w879 = 0.0 ("element")
        (unwired) 0.0 ("element")
        n356 = event-data() -> ("OldVal"=w909:bool)  [unwired: 1 in, 5 out]
        n357 = local write "Ende"(w909) -> ()
        n358 = local read "Datenspeicher"() -> (w880:T3)
        n359 = Unbundle By Name(w880) -> ("Rolle [Inkr/U]"=w901:u16, "Rollenumfang [m]"=w900:dbl, "Rollenträgheit [kgm²]"=w899:dbl, "Zündung [Imp/U]"=w898:dbl, "Getriebe [1:]"=w897:dbl, "Reifenumfang [m]"=w896:dbl, "Gl. Mittelwert"=w895:u8, "Differenzenquotient"=w894:u8, "Polynom"=w893:u8, "Lufttemperatur [°C]"=w892:dbl, "Luftfeuchtigkeit [%]"=w891:dbl, "Luftdruck [mbar]"=w889:dbl, "Best Polynomial Fit"=w890:dbl[], "Übersetzung ermitteln aus"=w888:u8, "[s]"=w887:dbl, "nmin [1/min]"=w886:dbl, "nmax [1/min]"=w885:dbl, "n vom Gas [1/min]"=w884:dbl, "Boolesch"=w883:bool, "Serielle Schnittstelle"=w878:refnum<visa-resource-name>)  [unwired: 3 out]
        n360 = call <vilib>:"Application Directory.vi"() -> ("Application Directory"=w906:path)
        n361 = Bundle By Name(cluster=w880, "Fahrzeugdaten"="", "date/time string"="", "Rolle [Inkr/U]"=w901, "Rollenumfang [m]"=w900, "Rollenträgheit [kgm²]"=w899, "Zündung [Imp/U]"=w898, "Getriebe [1:]"=w897, "Reifenumfang [m]"=w896, "element"=0.0, "Gl. Mittelwert"=w895, "Differenzenquotient"=w894, "Polynom"=w893, "element"=w879, "element"=w879, "Lufttemperatur [°C]"=w892, "Luftfeuchtigkeit [%]"=w891, "Luftdruck [mbar]"=w889, "Best Polynomial Fit"=w890, "Übersetzung ermitteln aus"=w888, "[s]"=w887, "nmin [1/min]"=w886, "nmax [1/min]"=w885, "n vom Gas [1/min]"=w884, "Boolesch"=w883, "Serielle Schnittstelle"=w878) -> (w881:T3)
        n362 = Build Path(base path=w906, name or relative path="Konfig.xml") -> (appended path=w904:path)
        n363 = Flatten To XML(anything=w881) -> (xml string=w908:string)
        n364 = call-poly <vilib>:"Write to XML File.vi"("XML Input"=w908, "XML File Path"=w904) -> ("error out"=w907:errorcluster)  [unwired: 7 in, 2 out]
        n365 = case shown="Kein Fehler" w907 {
          frame No Error {
          }
          frame Error {
          }
        }
      }
      event "Serielle Schnittstelle": Value Change {
        n366 = event-data() -> ()  [unwired: 1 in, 6 out]
        n367 = property on="Start" class="Bool. (strikt)"("DisabledEnum"=T4."Enabled" ("Deaktiviert")) -> ()  [unwired: 2 in, 2 out]
      }
      event "Messung Klimadaten": Value Change {
        n368 = event-data() -> ("NewVal"=w912:bool)  [unwired: 1 in, 5 out]
        n369 = case shown="True" w912 {
          frame True {
            w913 = T4."Disabled and Grayed Out" ("Deaktiviert")
            n370 = property on="Lufttemperatur [°C]" class="DigWert (strikt)"("DisabledEnum"=w913) -> ()  [unwired: 2 in, 2 out]
            n371 = property on="Luftdruck [mbar]" class="DigWert (strikt)"("DisabledEnum"=w913) -> ()  [unwired: 2 in, 2 out]
            n372 = property on="Luftfeuchtigkeit [%]" class="DigWert (strikt)"("DisabledEnum"=w913) -> ()  [unwired: 2 in, 2 out]
          }
          frame False {
            w914 = T4."Enabled" ("Deaktiviert")
            n373 = property on="Lufttemperatur [°C]" class="DigWert (strikt)"("DisabledEnum"=w914) -> ()  [unwired: 2 in, 2 out]
            n374 = property on="Luftdruck [mbar]" class="DigWert (strikt)"("DisabledEnum"=w914) -> ()  [unwired: 2 in, 2 out]
            n375 = property on="Luftfeuchtigkeit [%]" class="DigWert (strikt)"("DisabledEnum"=w914) -> ()  [unwired: 2 in, 2 out]
          }
        }
      }
      event "Recalc": Value Change {
        n376 = event-data() -> ("OldVal"=w917:bool)  [unwired: 1 in, 5 out]
        n377 = property on="Recalc" class="Bool. (strikt)"("Value"=w917) -> ()  [unwired: 2 in, 2 out]
        n378 = property on="Datenspeicher" class="Cluster (strikt)"() -> ("Value"=w915:T3)  [unwired: 2 in, 2 out]
        n379 = call "ReCalc_V2.00.vi"("Berechnen"=TRUE, "Datenspeicher"=w915) -> ()  [unwired: 3 in]
      }
      event "Übersetzung ermitteln aus": Value Change {
        n380 = event-data() -> ("NewVal"=w919:T2)  [unwired: 1 in, 5 out]
        n381 = case shown="\"nKuWe / nRolle\"" w919 {
          tunnel: [T4."Disabled and Grayed Out" ("Deaktiviert") T4."Disabled and Grayed Out" ("Deaktiviert") T4."Enabled" ("Deaktiviert")] -> w921
          frame "nKuWe / nRolle" {
          }
          frame "Zündsignal", Default {
          }
          frame "Getriebe & Reifen" {
          }
        }
        n382 = case shown="\"Zündsignal\", Standard" w919 {
          tunnel: [T4."Enabled" ("Deaktiviert") T4."Disabled and Grayed Out" ("Deaktiviert") T4."Disabled and Grayed Out" ("Deaktiviert")] -> w920
          frame "nKuWe / nRolle" {
          }
          frame "Zündsignal", Default {
          }
          frame "Getriebe & Reifen" {
          }
        }
        n383 = case shown="\"Zündsignal\", Standard" w919 {
          tunnel: [T4."Disabled and Grayed Out" ("Deaktiviert") T4."Enabled" ("Deaktiviert") T4."Disabled and Grayed Out" ("Deaktiviert")] -> w918
          frame "nKuWe / nRolle" {
          }
          frame "Zündsignal", Default {
          }
          frame "Getriebe & Reifen" {
          }
        }
        n384 = property on="Getriebe [1:]" class="DigWert (strikt)"("DisabledEnum"=w921) -> ()  [unwired: 2 in, 2 out]
        n385 = property on="Reifenumfang [m]" class="DigWert (strikt)"("DisabledEnum"=w921) -> ()  [unwired: 2 in, 2 out]
        n386 = property on="nKuWe/nRolle" class="DigWert (strikt)"("DisabledEnum"=w920) -> ()  [unwired: 2 in, 2 out]
        n387 = property on="Dauer [s]" class="DigWert (strikt)"("DisabledEnum"=w918) -> ()  [unwired: 2 in, 2 out]
        n388 = property on="Zündung [Imp/U]" class="DigWert (strikt)"("DisabledEnum"=w918) -> ()  [unwired: 2 in, 2 out]
      }
    }
    n389 = disable-structure shown="Deaktiviert" {
      disable-tunnel: w836 -> [w837 _]
      frame Disabled {
        n390 = Quit LabVIEW(quit? (T)=w837) -> ()
      }
      frame Enabled {
      }
    }
  }
